vi "Day 24 - Blizzard Basin.vi"() -> ()   [LabVIEW 2020, in "AoC 2022.lvlib"]
uses:
  AoC 2022.lvlib
  private/Valley Item.ctl
  Day 15 - Beacon Exclusion Zone/private/Location.ctl
  private/Valley Point.ctl
  ac79162b-5717-459b-9f1d-b916fa1d06b0.vi
panel:
  out "Active Elves":i32=100
  in  "Max Active Elves":i32=100
  out "FPS":dbl format="%#_3p"
  out "Puzzle Part-2 Answer":string
  out "Goal reaching Minutes":i32[](array[numeric])
  in  "millisecond multiple":u32=150
  out "#Minutes":i32
  in  "Visualizations":enum32{"Basic Real-Time", "Colorful Real-Time"}(tab)
  out "Valley (Basic)":string="#.######\n#>>.<^<#\n#.<..<<#\n#>v.><>#\n#<^v^^>#\n######.#"
  out "Valley (Colorful)":u32[][](array[colorbox])
  out "Colors":u32[](array[colorbox])
  out "Legend":T1[](array[typedef])=[enum."#", enum.".", enum.">", enum."<", enum."^", enum."v", enum."E"]
  in  "Puzzle Input":string="#.######\n#>>.<^<#\n#.<..<<#\n#>v.><>#\n#<^v^^>#\n######.#"
  out "Puzzle Answer":string
  # "Press Ctrl+M & Enter the Puzzle Input and run the VI"
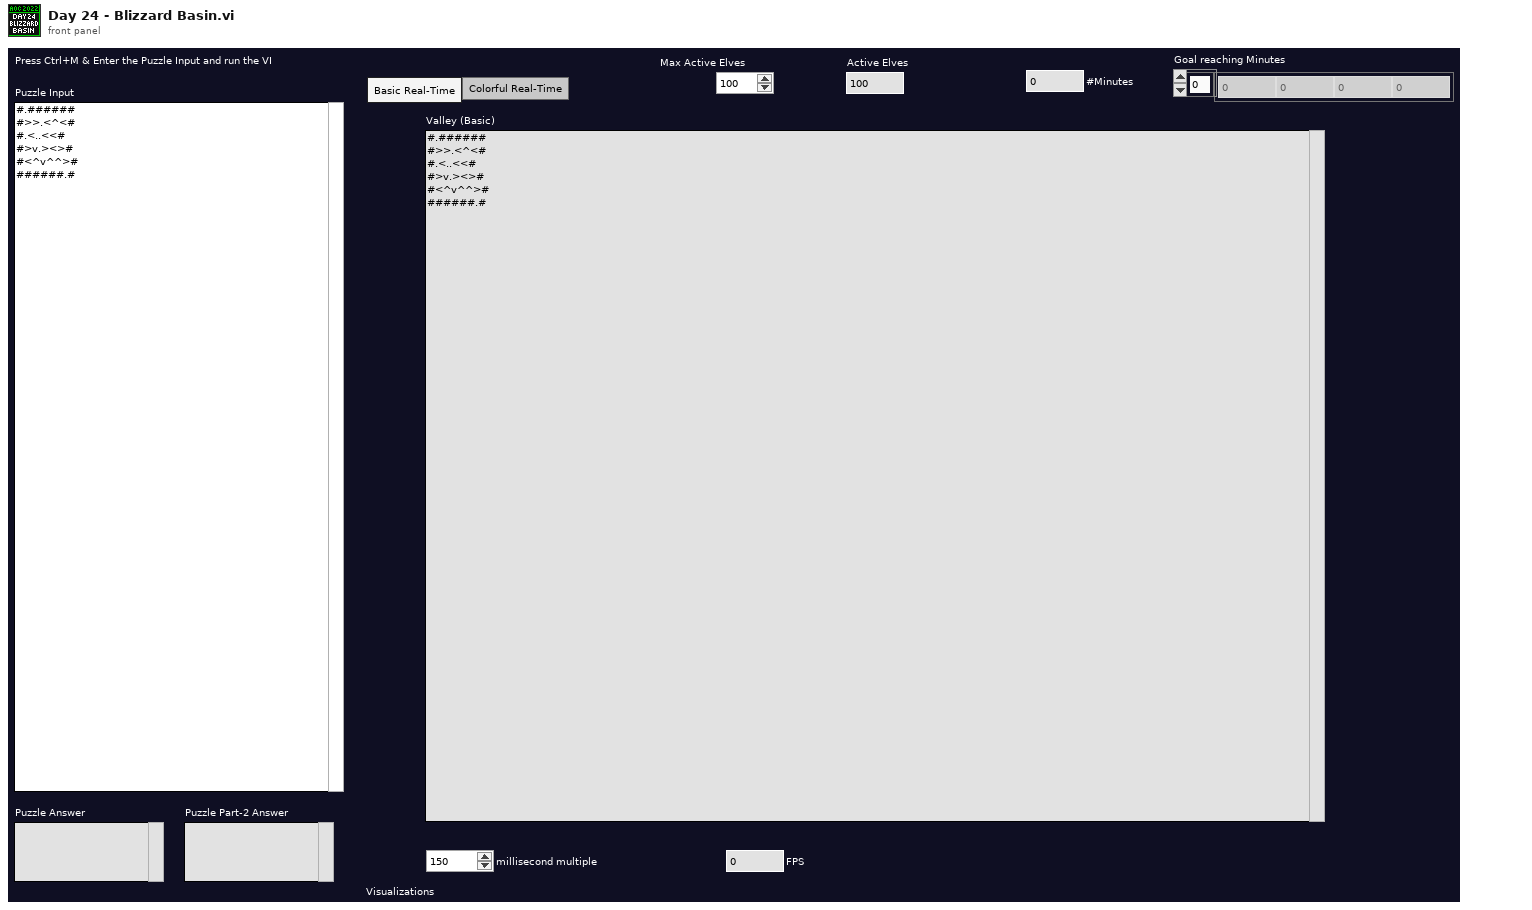
[diagram p1: front panel]
types:
  T1 = typedef "AoC 2022.lvlib/Valley Item.ctl" = enum16{"#", ".", ">", "<", "^", "v", "E"}
  T2 = typedef "AoC 2022.lvlib/Valley Point.ctl" = cluster{"Items":T1[]}
  T3 = typedef "AoC 2022.lvlib/Location.ctl" = cluster{"X":i32, "Y":i32}
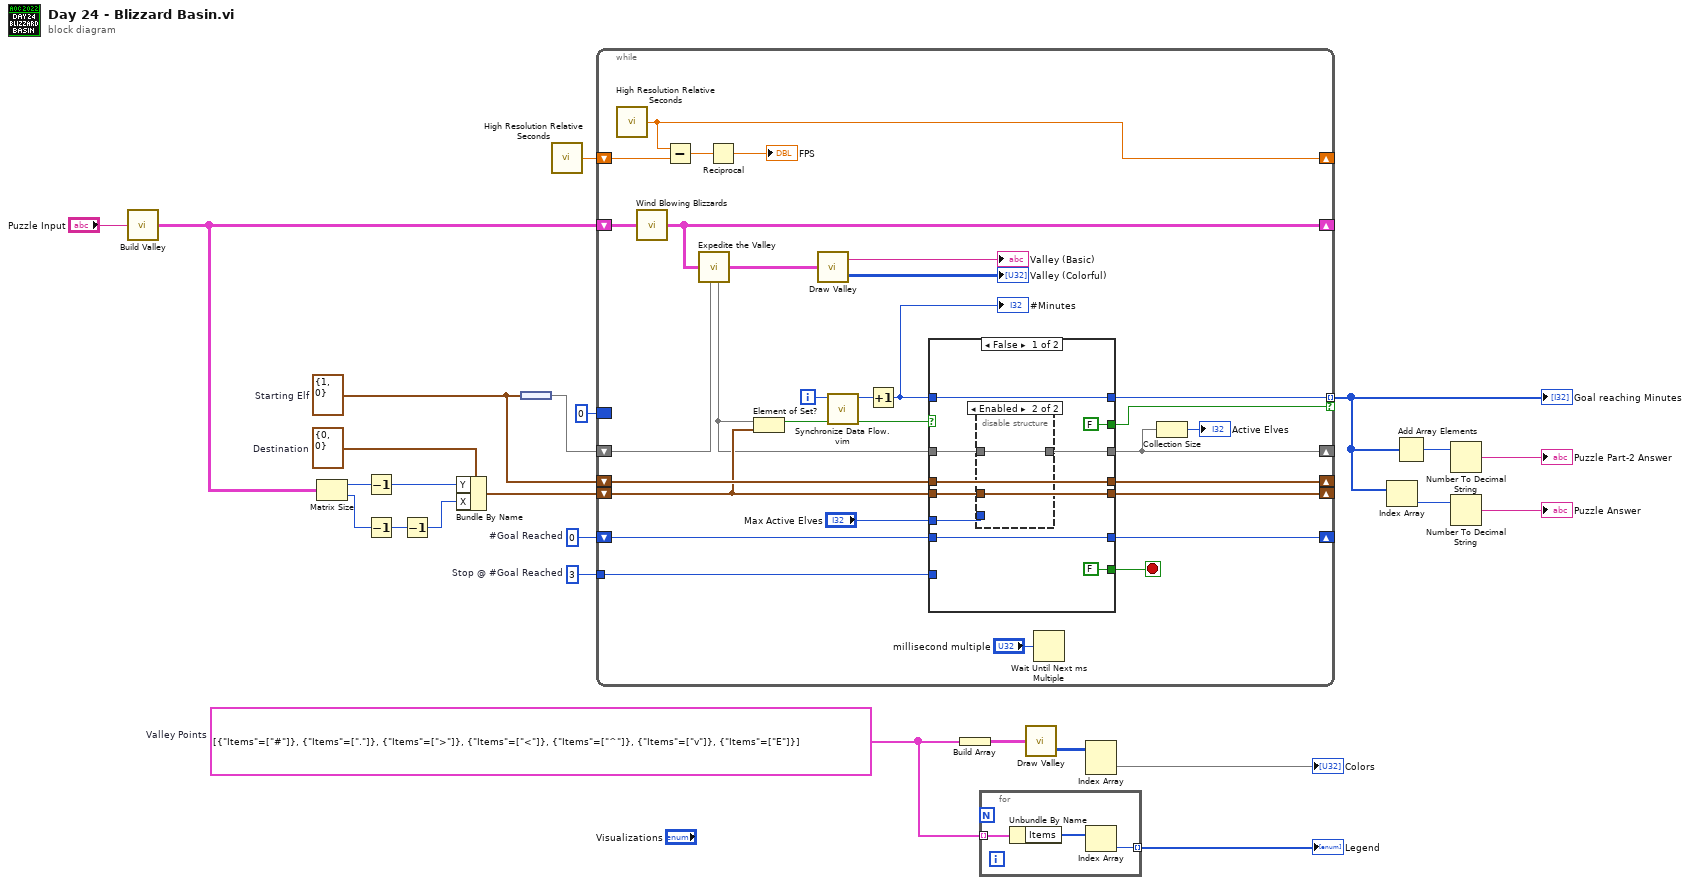
[diagram p0: block diagram]
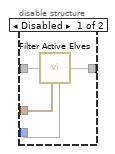
[diagram p2: hidden frame]
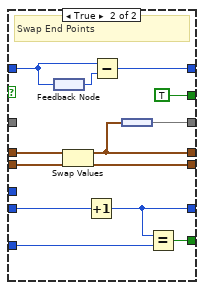
[diagram p3: hidden frame]
diagram:
  w4 = T2[] [{"Items"=[enum."#"]}, {"Items"=[enum."."]}, {"Items"=[enum.">"]}, {"Items"=[enum."<"]}, {"Items"=[enum."^"]}, {"Items"=[enum."v"]}, {"Items"=[enum."E"]}]  # Valley Points
  w14 = 3  # Stop @ #Goal Reached
  w13 = 0  # #Goal Reached
  w19 = T3 {"X"=0, "Y"=0}  # Destination
  w15 = T3 {"X"=1, "Y"=0}  # Starting Elf
  n1 = call "Build Valley.vi"("Puzzle Input"="Puzzle Input") -> ("Valley"=w23:T2[][])
  n2 = Matrix Size(0:w23) -> (1:w22:i32, 2:w21:i32)
  n3 = Decrement(x=w22) -> (x-1=w18:i32)
  n4 = Decrement(x=w21) -> (x-1=w20:i32)
  n5 = Decrement(x=w20) -> (x-1=w17:i32)
  n6 = Bundle By Name(cluster=w19, "Y"=w18, "X"=w17) -> (w16:T3)
  n7 = node(w15) -> (w24:set{T3})
  n8 = call <vilib>:"High Resolution Relative Seconds.vi"() -> ("relative seconds"=w1:dbl)
  n9 = while {
    shift-right: [w52] -> _
    shift-left: w23 -> [w55]
    shift-right: [w27] -> _
    shift-left: w24 -> [w53]
    shift-right: [w41] -> _
    shift-left: w16 -> [w43]
    shift-right: [w42] -> _
    shift-left: w15 -> [w44]
    shift-right: [w40] -> _
    shift-left: w13 -> [w39]
    tunnel: [w36] -> w9 mode=indexing if=w35
    tunnel: w14 -> [w47]
    border: 0 -> [_]
    shift-right: [w33] -> _
    shift-left: w1 -> [w34]
    i -> [w49]
    stop <- w46 stop-if-true
    n10 = call <vilib>:"High Resolution Relative Seconds.vi"() -> ("relative seconds"=w33:dbl)
    n11 = call "Wind Blowing Blizzards.vi"("Valley in"=w55) -> ("Valley out"=w52:T2[][])
    n12 = Subtract(x=w33, y=w34) -> (x-y=w32:dbl)
    n13 = call "Expedite the Valley.vi"("Valley in"=w52, "Elf Locations in"=w53) -> ("Elf Locations out"=w38:set{T3}, "Valley out"=w54:T2[][])
    n14 = Reciprocal(x=w32) -> (1/x=→"FPS":dbl)
    n15 = Element of Set?(10:w43, 11:w38) -> (3:w50:bool)
    n16 = call "Draw Valley.vi"("Valley Points"=w54) -> ("Valley Basic"=→"Valley (Basic)":string, "Valley Colorful"=→"Valley (Colorful)":u32[][])
    n17 = call "Synchronize Data Flow.vim"("input 4"=w50, "input 1"=w49) -> ("output 4"=w45:bool, "output 1"=w48:i32)  [unwired: 2 in, 2 out]
    n18 = Increment(x=w48) -> (x+1=w37:i32)
    "#Minutes" <- w37
    n19 = case shown="False" w45 {
      tunnel: w47 -> [_ w82]
      tunnel: [FALSE w81] -> w46
      tunnel: w44 -> [w64 w80]
      tunnel: w43 -> [w57 w79]
      tunnel: [w64 w76] -> w42
      tunnel: [w57 w78] -> w41
      tunnel: [w63 w74] -> w40
      tunnel: w39 -> [w63 w75]
      tunnel: w38 -> [w59 _]
      tunnel: [w58 w77] -> w27
      tunnel: w37 -> [w61 w73]
      tunnel: [w61 w71] -> w36
      tunnel: [FALSE TRUE] -> w35
      tunnel: "Max Active Elves" -> [w56 _]
      frame False {
        n20 = disable-structure shown="Enabled" {
          disable-tunnel: w59 -> [w68 w69]
          disable-tunnel: [w67 w69] -> w58
          disable-tunnel: w57 -> [w66 _]
          disable-tunnel: w56 -> [w65 _]
          frame Disabled {
            n21 = call "Filter Active Elves.vi"("Elf Locations in"=w68, "Destination"=w66, "#Active Elves"=w65) -> ("Elf Locations out"=w67:set{T3})
          }
          frame Enabled {
          }
        }
      }
      frame True {
        # "Swap End Points"
        n22 = feedback #1() -> (w72:i32)
        n23 = feedback-in #1(w73) -> ()
        n24 = Swap Values(12:w80, 14:w79) -> (1:w76:T3, 3:w78:T3)  [unwired: 1 in]
        n25 = Increment(x=w75) -> (x+1=w74:i32)
        n26 = Subtract(x=w73, y=w72) -> (x-y=w71:i32)
        n27 = node(w76) -> (w77:set{T3})
        n28 = Equal?(x=w74, y=w82) -> (x = y?=w81:bool)
      }
    }
    n29 = Wait Until Next ms Multiple(millisecond multiple="millisecond multiple") -> ()  [unwired: 1 out]
    n30 = Collection Size(1:w27) -> (0:→"Active Elves":i32)
  }
  "Goal reaching Minutes" <- w9
  n31 = Build Array(w4) -> (w3:T2[][])
  n32 = for {
    tunnel: w4 -> [w85] mode=indexing
    tunnel: [w83] -> w2 mode=indexing
    n33 = Unbundle By Name(w85) -> ("Items"=w84:T1[])
    n34 = Index Array(array=w84) -> (element=w83:T1)  [unwired: 1 in]
  }
  "Legend" <- w2
  n35 = call "Draw Valley.vi"("Valley Points"=w3) -> ("Valley Colorful"=w6:u32[][])  [unwired: 1 out]
  n36 = Index Array(array=w6) -> (element=→"Colors":u32[])  [unwired: 2 in]
  n37 = Index Array(array=w9) -> (element=w11:i32)  [unwired: 1 in]
  n38 = Add Array Elements(numeric array=w9) -> (sum=w8:i32)
  n39 = Number To Decimal String(number=w8) -> (decimal integer string=→"Puzzle Part-2 Answer":string)  [unwired: 1 in]
  n40 = Number To Decimal String(number=w11) -> (decimal integer string=→"Puzzle Answer":string)  [unwired: 1 in]
